vi "StartIfCan.vi"(11 "In Task":T1) -> (3 "Out Task":T1)   [LabVIEW 2012]
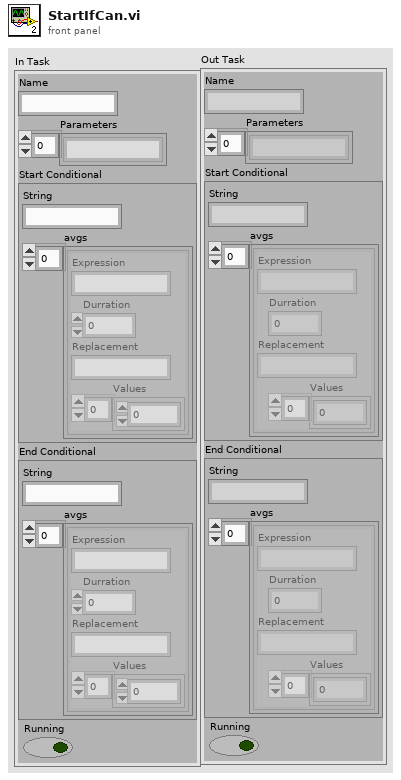
[diagram p1: front panel]
types:
  T1 = cluster{"Name":string, "Parameters":string[], "Start Conditional":cluster{"String":string, "avgs":cluster{"Expression":string, "Durration":dbl, "Replacement":string, "Values":dbl[]}[]}, "End Conditional":cluster{"String":string, "avgs":cluster{"Expression":string, "Durration":dbl, "Replacement":string, "Values":dbl[]}[]}, "Running":bool}
  T2 = cluster{"String":string, "avgs":cluster{"Expression":string, "Durration":dbl, "Replacement":string, "Values":dbl[]}[]}
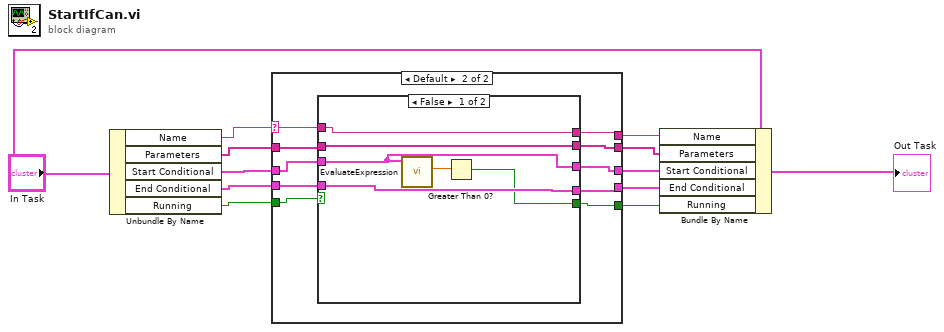
[diagram p0: block diagram]
diagram:
  n1 = Unbundle By Name("In Task") -> ("Name"=w7:string, "Parameters"=w9:string[], "Start Conditional"=w8:T2, "End Conditional"=w10:T2, "Running"=w6:bool)
  n2 = case shown="Default" w7 {
    selector: w7 -> [w16 w20]
    tunnel: w10 -> [w13 w24]
    tunnel: w9 -> [w15 w21]
    tunnel: w8 -> [w14 w25]
    tunnel: [w17 w26] -> w1
    tunnel: w6 -> [w17 w27]
    tunnel: [w16 w19] -> w5
    tunnel: [w15 w22] -> w4
    tunnel: [w14 w18] -> w3
    tunnel: [w13 w23] -> w2
    frame "None" {
    }
    frame Default {
      n3 = case shown="False" w27 {
        selector: w27 -> [_ w38]
        tunnel: [w29 w38] -> w26
        tunnel: w25 -> [w28 w36]
        tunnel: w24 -> [w33 w37]
        tunnel: [w33 w37] -> w23
        tunnel: [w28 w36] -> w18
        tunnel: w21 -> [w32 w35]
        tunnel: [w32 w35] -> w22
        tunnel: w20 -> [w31 w34]
        tunnel: [w31 w34] -> w19
        frame False {
          n4 = call "EvaluateExpression.vi"("Parsed Expression"=w28) -> ("Result"=w30:dbl)  [unwired: 9 in, 1 out]
          n5 = Greater Than 0?(x=w30) -> (x > 0?=w29:bool)
        }
        frame True {
        }
      }
    }
  }
  n6 = Bundle By Name(cluster="In Task", "Name"=w5, "Parameters"=w4, "Start Conditional"=w3, "End Conditional"=w2, "Running"=w1) -> (→"Out Task":T1)
